vi "FTW-ActorContext-InitializeBroker.vi"(0 "Actor Context":refnum<class "FTW-Actor-Context.lvclass">, 11 "error in":errorcluster) -> (4 "Actor Context out":refnum<class "FTW-Actor-Context.lvclass">, 15 "error out":errorcluster)   [LabVIEW 2013, in "FTW-Actor-Context.lvclass"]
uses:
  FTW-Actor-Context.lvclass
  FTW-Actor-Context.lvclass/FTW-Actor-Context.ctl
  Messaging/Broker/FTW-Actor-Broker.lvclass
panel:
  # "Inputs"
  # "Outputs"
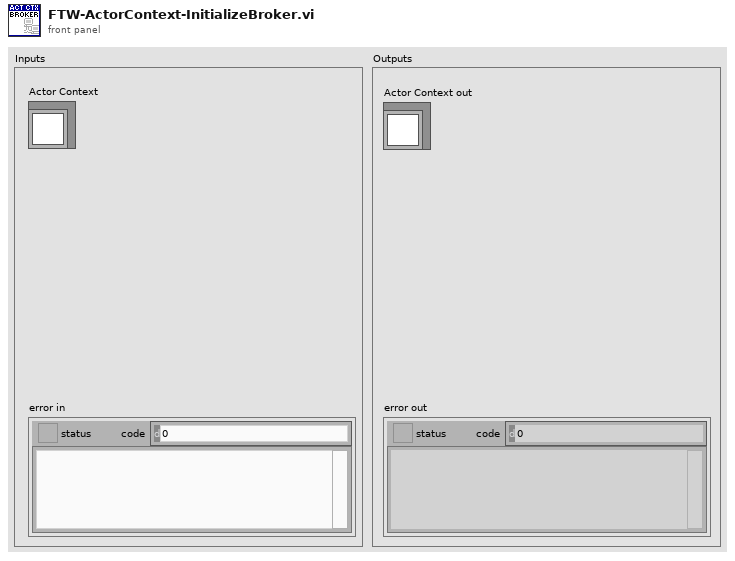
[diagram p1: front panel]
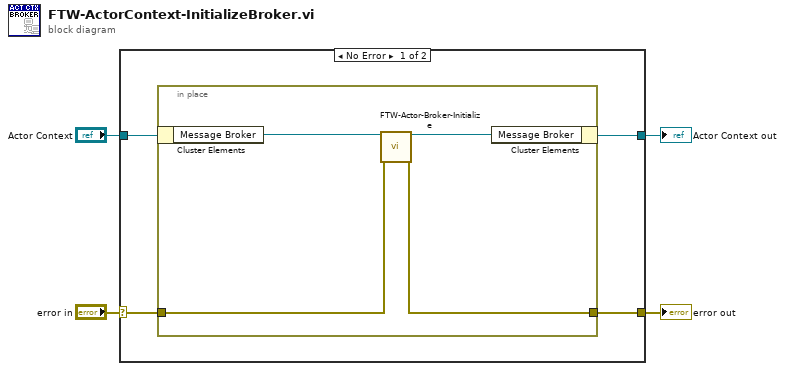
[diagram p0: block diagram]
diagram:
  n1 = case shown="No Error" "error in" {
    selector: "error in" -> [w7 w14]
    tunnel: [w6 w14] -> w4
    tunnel: [w5 w13] -> w2
    tunnel: "Actor Context" -> [w8 w13]
    frame No Error {
      n2 = in-place {
        in-place-border: w7 -> [w10]
        in-place-border: [w9] -> w6
        n3 = in-place-cluster #1(w8) -> ("Message Broker"=w12:refnum<class "FTW-Actor-Broker.lvclass">)
        n4 = call "FTW-Actor-Broker-Initialize.vi"("FTW Message Broker"=w12, "error in"=w10) -> ("FTW Message Broker out"=w11:refnum<class "FTW-Actor-Broker.lvclass">, "error out"=w9:errorcluster)  [unwired: 11 in, 1 out]
        n5 = in-place-cluster #1("Message Broker"=w11) -> (w5:refnum<class "FTW-Actor-Context.lvclass">)
      }
    }
    frame Error {
    }
  }
  "error out" <- w4
  "Actor Context out" <- w2
